vi "mlink_ao_scan_stop.vi"(8 "error in (no error)":errorcluster, 11 "connection ID":i32=-1) -> (0 "error out":errorcluster, 3 "connection ID out":i32)   [LabVIEW 2009, in "MicroDAQ.lvlib" / "mlink.lvlib"]
doc: "This function stops analog output scanning session. Function can be used to interrupt acquisition (duration > 0), or to stop continuous acquisition (duration=-1). After calling mlink_ao_scan_stop() function, scanning session has to be re-initialized."
uses:
  <instrlib>/MicroDAQ/Mlink library wraper/mlink.lvlib
  <instrlib>/MicroDAQ/MLink32.dll
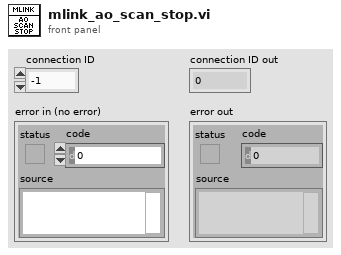
[diagram p1: front panel]
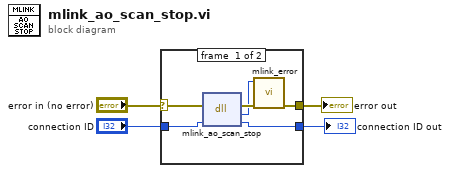
[diagram p0: block diagram]
diagram:
  n1 = case shown="No Error" "error in (no error)" {
    selector: "error in (no error)" -> [w10 w12]
    tunnel: [w9 w11] -> w3
    tunnel: "connection ID" -> [w8 w11]
    tunnel: [w5 w12] -> w1
    frame #0 {
      n2 = dll-call lib="C:/Program Files (x86)/National Instruments/LabVIEW 2009/instr.lib/MicroDAQ/MLink32.dll" fn="mlink_ao_scan_stop"(error in=w10, "connection ID"=w8) -> (error out=w7:errorcluster, "return type"=w6:i32, "connection ID"=w9:i32)  [unwired: 2 in, 1 out]
      n3 = call <instrlib>:"mlink_error.vi"("error in (no error)"=w7, "error code"=w6) -> ("error out"=w5:errorcluster)  [unwired: 9 in]
    }
    frame #1 {
    }
  }
  "error out" <- w1
  "connection ID out" <- w3
